vi "SMO.Example.About.vi"(8 "error in (no error)":errorcluster, 11 "SMO.Example":refnum<class "SMO.Example.lvclass">) -> (0 "error out":errorcluster, 3 "SMO.Example out":refnum<class "SMO.Example.lvclass">)   [LabVIEW 2013, in "SMO.Example.lvclass"]
doc: "---------------------------------------------------------------\nJKI State Machine Objects™\nhttp://jki.net/state-machine-objects/\nCopyright (C) 2005-2015, JKI <info@jki.net>\nALL RIGHTS RESERVED"
uses:
  SMO.Example.lvclass
  SMO.UI/SMO.UI.lvclass
panel:
  # "For instructions on how to use the JKI State Machine Objects, examples and video tutorials, visit:\nhttp://jki.net/state-machine-objects/\n\nJKI State Machine Objects™\nhttp://jki.net/state-machine-objects/\nCopyright (C) 2005-2015, JKI <info@jki.net>\nALL RIGHTS RESERVED"
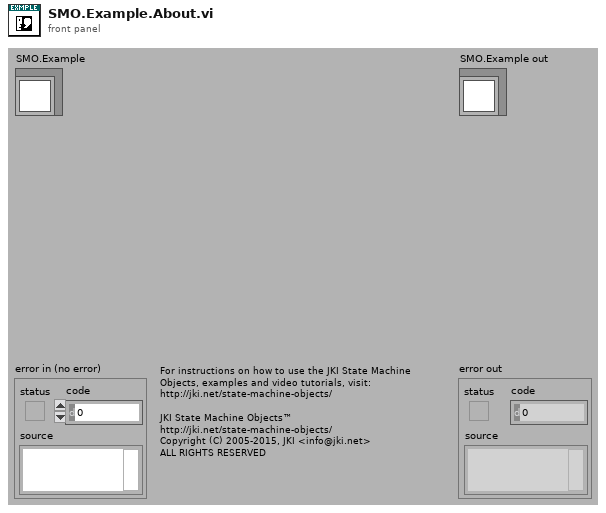
[diagram p1: front panel]
types:
  T1 = typedef "SMO.Example.lvclass/Dependencies--Cluster.ctl" = cluster{"About":refnum<class "SMO.UI.lvclass">}
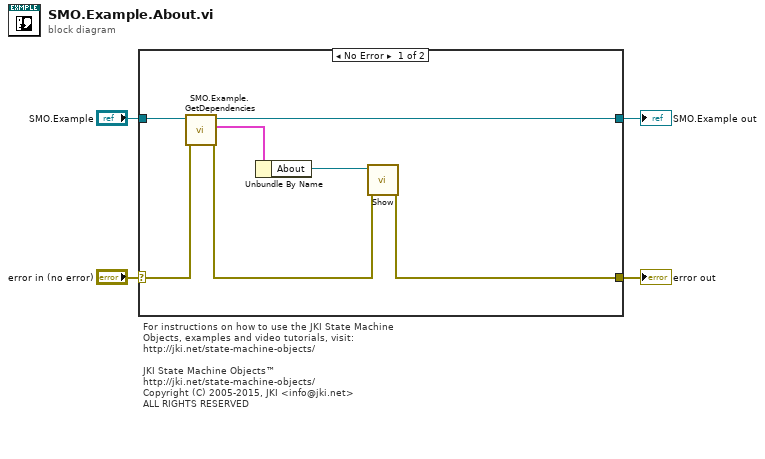
[diagram p0: block diagram]
diagram:
  # "For instructions on how to use the JKI State Machine Objects, examples and video tutorials, visit:\nhttp://jki.net/state-machine-objects/\n\nJKI State Machine Objects™\nhttp://jki.net/state-machine-objects/\nCopyright (C) 2005-2015, JKI <info@jki.net>\nALL RIGHTS RESERVED"
  n1 = case shown="No Error" "error in (no error)" {
    selector: "error in (no error)" -> [w10 w12]
    tunnel: "SMO.Example" -> [w11 w13]
    tunnel: [w5 w12] -> w3
    tunnel: [w9 w13] -> w2
    frame No Error {
      n2 = call "SMO.Example.GetDependencies.vi"("error in (no error)"=w10, "SMO.Example"=w11) -> ("error out"=w6:errorcluster, "Dependencies"=w8:T1, "SMO.Example out"=w9:refnum<class "SMO.Example.lvclass">)  [unwired: 7 in]
      n3 = Unbundle By Name(w8) -> ("About"=w7:refnum<class "SMO.UI.lvclass">)
      n4 = call "Show.vi"("error in (no error)"=w6, "SMO.UI"=w7) -> ("error out"=w5:errorcluster)  [unwired: 8 in, 1 out]
    }
    frame Error {
    }
  }
  "error out" <- w3
  "SMO.Example out" <- w2
